vi "set clear fault.vi"(8 "error in (no error)":errorcluster, 11 "Cobolt in":refnum<class "Cobolt.lvclass">) -> (0 "error out":errorcluster, 3 "Cobolt out":refnum<class "Cobolt.lvclass">)   [LabVIEW 2012, in "Cobolt.lvclass"]
uses:
  Cobolt.lvclass
  CoboltLaserDrivers_Public_LV2012/CoboltLaser_Controls/ExpectedResponseType.ctl
  Cobolt.lvclass/Cobolt.ctl
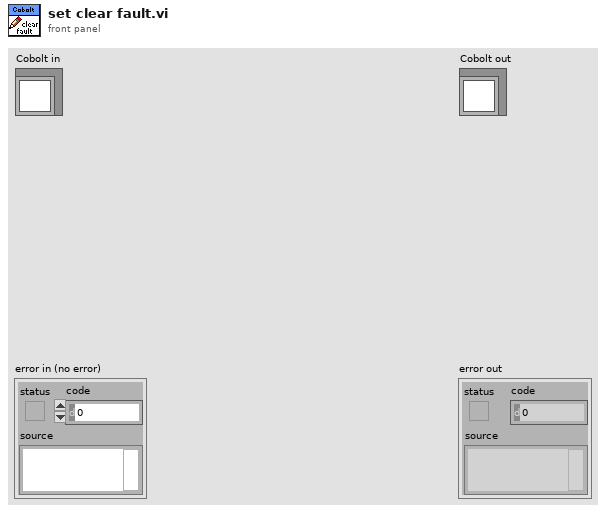
[diagram p1: front panel]
types:
  T1 = typedef "Cobolt.lvclass/ExpectedResponseType.ctl" = u16
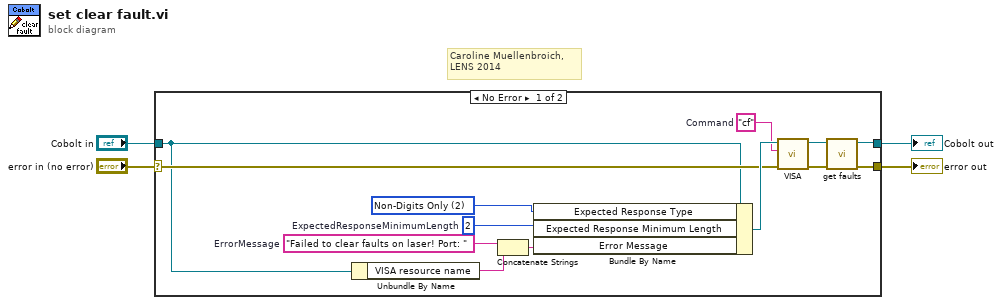
[diagram p0: block diagram]
diagram:
  # "Caroline Muellenbroich, \nLENS 2014"
  n1 = case shown="No Error" "error in (no error)" {
    selector: "error in (no error)" -> [w11 w19]
    tunnel: [w5 w19] -> w3
    tunnel: [w6 w18] -> w1
    tunnel: "Cobolt in" -> [w10 w18]
    frame No Error {
      w9 = "cf"  # Command
      w12 = T1 2 items=["Any", "Digits Only", "Non-Digits Only"] ("ExpectedResponseType")
      w16 = 2  # ExpectedResponseMinimumLength
      w14 = "Failed to clear faults on laser! Port: "  # ErrorMessage
      n2 = Unbundle By Name(w10) -> ("VISA resource name"=w15:string)
      n3 = Concatenate Strings(w14, w15) -> (w13:string)
      n4 = Bundle By Name(cluster=w10, "Expected Response Type"=w12, "Expected Response Minimum Length"=w16, "Error Message"=w13) -> (w17:refnum<class "Cobolt.lvclass">)
      n5 = call-dynamic "VISA.vi"("error in (no error)"=w11, "string to write"=w9, "Cobolt in"=w17) -> ("error out"=w8:errorcluster, "Cobolt out"=w7:refnum<class "Cobolt.lvclass">)  [unwired: 6 in, 1 out]
      n6 = call-dynamic "get faults.vi"("error in (no error)"=w8, "Cobolt in"=w7) -> ("error out"=w5:errorcluster, "Cobolt out"=w6:refnum<class "Cobolt.lvclass">)  [unwired: 8 in]
    }
    frame Error {
    }
  }
  "error out" <- w3
  "Cobolt out" <- w1
